vi "WPGraph.vi"(9 "History Buffers":T1, 10 "Ring Buffers":T1) -> (0 "Last Points":dbl[](array[numeric]), 1 "Latest Points":cluster{dbl[], dbl[]}[](graph), 2 "History Buffer":dbl[][](graph), 3 "Ring Buffer":cluster{dbl[], dbl[]}[](graph))   [LabVIEW 2017, in "Collection.lvclass"]
doc: "Unpacks the ring and history buffers of a collection array and plots the points from each time against each other."
uses:
  Collection.lvclass
  Readable/TX Graph.ctl
  Readable/Readable.lvclass
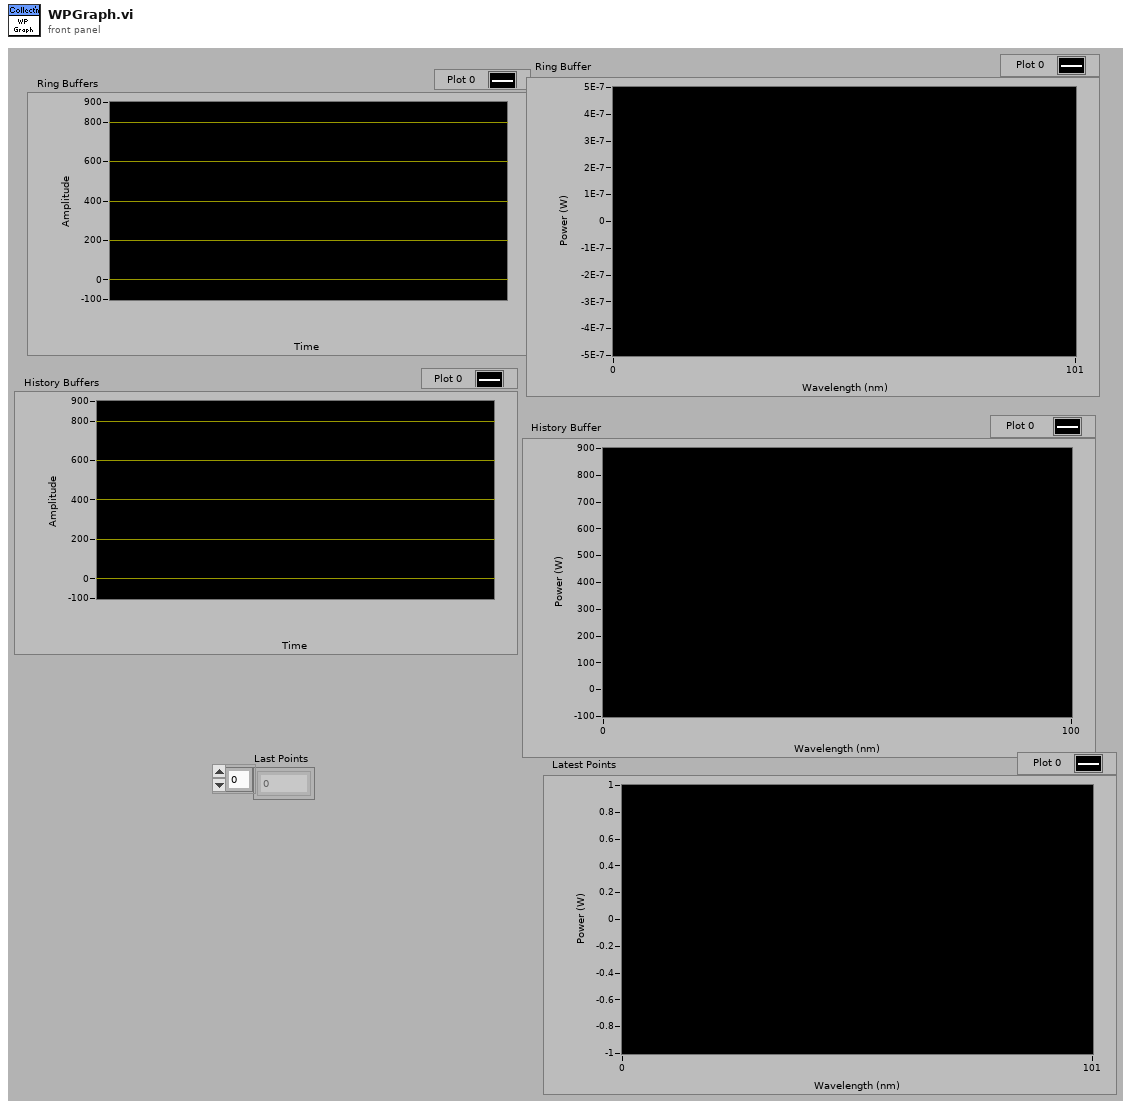
[diagram p1: front panel]
types:
  T1 = typedef "Readable.lvclass/TX Graph.ctl" = cluster{"Data Points":cluster{"t":timestamp, "x":dbl}[]}[]
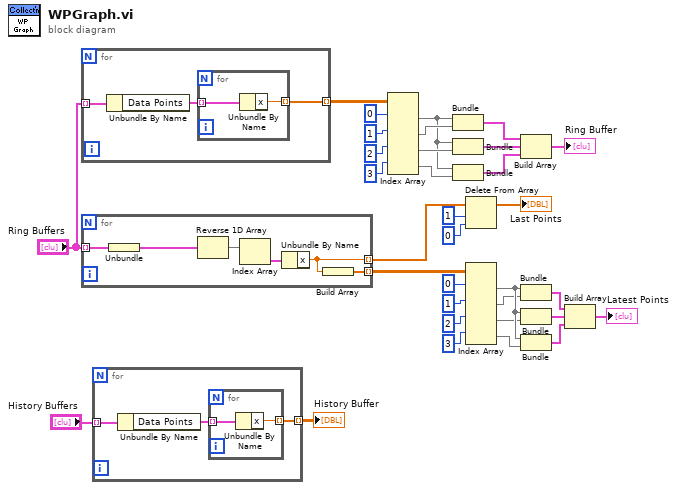
[diagram p0: block diagram]
diagram:
  n1 = for {
    tunnel: [w35] -> w24 mode=indexing
    tunnel: "Ring Buffers" -> [w34] mode=indexing
    n2 = Unbundle By Name(w34) -> ("Data Points"=w36:cluster{"t":timestamp, "x":dbl}[])
    n3 = for {
      tunnel: w36 -> [w38] mode=indexing
      tunnel: [w37] -> w35 mode=indexing
      n4 = Unbundle By Name(w38) -> ("x"=w37:dbl)
    }
  }
  n5 = for {
    tunnel: "Ring Buffers" -> [w43] mode=indexing
    tunnel: [w40] -> w5 mode=indexing
    tunnel: [w39] -> w2 mode=indexing
    n6 = Unbundle(w43) -> ("Data Points"=w42:cluster{"t":timestamp, "x":dbl}[])
    n7 = Reverse 1D Array(array=w42) -> (reversed array=w41:cluster{"t":timestamp, "x":dbl}[])
    n8 = Index Array(array=w41) -> (element=w44:cluster{"t":timestamp, "x":dbl})  [unwired: 1 in]
    n9 = Unbundle By Name(w44) -> ("x"=w39:dbl)
    n10 = Build Array(w39) -> (w40:dbl[])
  }
  n11 = for {
    tunnel: "History Buffers" -> [w47] mode=indexing
    tunnel: [w45] -> w32 mode=indexing
    n12 = Unbundle By Name(w47) -> ("Data Points"=w46:cluster{"t":timestamp, "x":dbl}[])
    n13 = for {
      tunnel: w46 -> [w49] mode=indexing
      tunnel: [w48] -> w45 mode=indexing
      n14 = Unbundle By Name(w49) -> ("x"=w48:dbl)
    }
  }
  "History Buffer" <- w32
  n15 = Index Array(array=w24, index (row) #1=0 ("disabled index (col)"), index (row) #2=1 ("index (col)"), index (row) #3=2 ("index (col)"), index (row) #4=3 ("index (col)")) -> (element #1=w29:dbl[], element #2=w31:dbl[], element #3=w30:dbl[], element #4=w28:dbl[])  [unwired: 4 in]
  n16 = Bundle(w29, w31) -> (w27:cluster{dbl[], dbl[]})  [unwired: 1 in]
  n17 = Bundle(w29, w30) -> (w26:cluster{dbl[], dbl[]})  [unwired: 1 in]
  n18 = Bundle(w29, w28) -> (w25:cluster{dbl[], dbl[]})  [unwired: 1 in]
  n19 = Delete From Array(array=w2, length=1, index=0 ("index (row)")) -> (array with subset deleted=→"Last Points":dbl[])  [unwired: 1 out]
  n20 = Index Array(array=w5, index (row) #1=0 ("disabled index (col)"), index (row) #2=1 ("index (col)"), index (row) #3=2 ("index (col)"), index (row) #4=3 ("index (col)")) -> (element #1=w14:dbl[], element #2=w6:dbl[], element #3=w13:dbl[], element #4=w12:dbl[])  [unwired: 4 in]
  n21 = Build Array(w27, w26, w25) -> (→"Ring Buffer":cluster{dbl[], dbl[]}[])
  n22 = Bundle(w14, w6) -> (w11:cluster{dbl[], dbl[]})  [unwired: 1 in]
  n23 = Bundle(w14, w13) -> (w10:cluster{dbl[], dbl[]})  [unwired: 1 in]
  n24 = Bundle(w14, w12) -> (w9:cluster{dbl[], dbl[]})  [unwired: 1 in]
  n25 = Build Array(w11, w10, w9) -> (→"Latest Points":cluster{dbl[], dbl[]}[])
